vi "GetType.vi"(8 "error in (no error)":errorcluster, 11 "Configure Power Line Frequency [PLF] Msg":refnum<class "Configure Power Line Frequency [PLF] Msg.lvclass">) -> (0 "error out":errorcluster, 2 "Data Sample":variant, 3 "Configure Power Line Frequency [PLF] Msg":refnum<class "Configure Power Line Frequency [PLF] Msg.lvclass">)   [LabVIEW 2016, in "CS++DMM.lvlib" / "Configure Power Line Frequency [PLF] Msg.lvclass"]
uses:
  Configure Power Line Frequency [PLF] Msg.lvclass
  Configure Power Line Frequency [PLF] Msg.lvclass/Configure Power Line Frequency [PLF] Msg.ctl
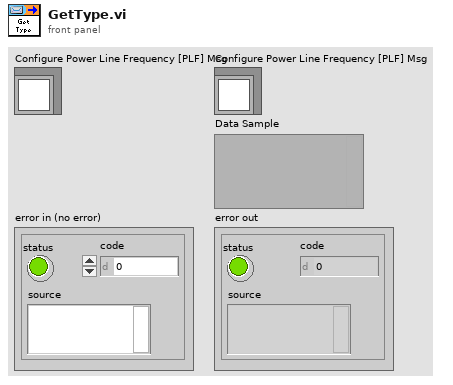
[diagram p1: front panel]
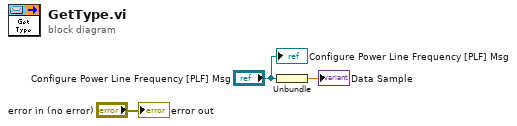
[diagram p0: block diagram]
diagram:
  n1 = Unbundle("Configure Power Line Frequency [PLF] Msg") -> (→"Data Sample":dbl)
  "error out" <- "error in (no error)"
  "Configure Power Line Frequency [PLF] Msg" <- "Configure Power Line Frequency [PLF] Msg"
